vi "CRYPreLoad Project.vi"(4 "Only create refnums (F)":bool) -> ()   [LabVIEW 2013]
uses:
  CRYMainGlobal.vi
  CRYProject Editor Global.vi
  CRYSystem/Program/CRYRef nums global.vi
  CRYSystem/Task Sequence/CRYProject Run Control Global.vi
panel:
  in  "VISA serial ports (empty array)":T1(array[cluster]) {"COM port (1 = COM1, etc.)" min=1 max=99}
  in  "VISA session (for class)":refnum<visa-resource-name>
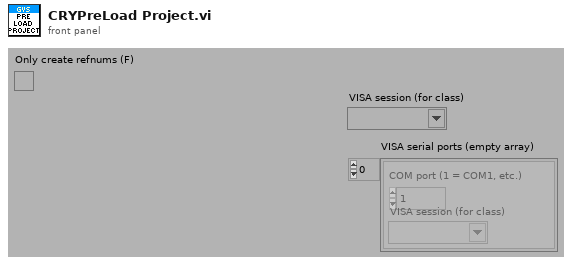
[diagram p1: front panel]
types:
  T1 = cluster{"COM port (1 = COM1, etc.)":i32, "VISA session (for class)":refnum<visa-resource-name>}[]
  T2 = typedef "CRYTS.ctl" = cluster{"No.TS":u16, "TS File Path":path, "TS Name":string, "EditStepName":string, "Steps":T3[], "New State":bool, "Change State":bool, "Flattened CurveLib Data":string, "Document Data":string, "EditStepNo":u16, "Operator Start File":string, "Sequence Type":string, "Sequence Language":string}
  T3 = typedef "CRYStep.ctl" = cluster{"No.VI":i32, "Category":string, "StepName":string, "Seq setup flattened":string, "Comment":string, "Steps config.":bool[], "Jump config":i32[], "Start":dbl, "Increment":dbl, "Name":string, "Unit":string, "Y data":u16, "Y prefix":string, "Y dB ref":dbl, "Y unit":string, "Repeat State Array":cluster{"Start":dbl, "Increment":dbl, "Count":i32, "Num":i32}[]}
  T4 = typedef "CRYHardware.ctl" = cluster{"Name":string, "Analog I/O":u16, "Digital I/O":u16, "Channels":u8, "Dig Dev ID":u8, "N ports":u8, "Interface":u32, "Dig I/O Ports":cluster{"port #":i16, "width":i16, "direction":i32}[], "Interf settings":cluster{"Type":u16, "COM Port":u8, "Baud rate":u32, "Data bits":u32, "Parity":u16, "Stop bits":u16, "Flow control":u16, "Dev ID IEEE":u8}[], "N interfs":i32, "udev SNs":i16[], "udev enable":bool, "Channel Array":T5[], "Cal sequence":string, "SelectedIn":u16, "SelectedOut":u16, "SelectedTab":u16, "State":bool, "Help":string, "Advanced":bool, "In Audio Driver":u16, "Out Audio Driver":u16}
  T5 = typedef "CRYHardware Channel Info.ctl" = cluster{"ID":i32, "Name":string, "Digital":bool, "Input":bool, "Device Name":string, "Hardware Ch ID":u8, "Vmax (V)":dbl, "Latency (samples)":dbl, "Sampling Rate (Hz)":u32, "Bit Depth":u32, "Anti-aliasing Factor (%fs)":sgl, "DAQmx Channel":tag, "term config":i32, "Coupling":i32, "IEPE en":bool, "ASIOChannel Name":string, "Audio Driver":u16, "ASIOChannel Index":u8}
  T6 = cluster{"port #":i16, "width":i16, "direction":i32}[]
  T7 = cluster{"Type":u16, "COM Port":u8, "Baud rate":u32, "Data bits":u32, "Parity":u16, "Stop bits":u16, "Flow control":u16, "Dev ID IEEE":u8}[]
  T8 = typedef "CRYStart Cluster.ctl" = cluster{"SequenceName":string, "Preload Stimulus":bool, "CloseOpenedDisplay":bool, "ClearMeasuredData":bool, "UpdateDisplayDuringRun":bool, "DisplayForConfirmation":bool, "HaltOnFail":bool, "UseSameHardware":bool, "UseSameCalibration":bool}
  T9 = cluster{"DIO Port Config":refnum<vi>, "DIO Port Write":refnum<vi>, "DIO Port Read":refnum<vi>}
  T10 = cluster{"input XON/XOFF":bool, "input HW Handshake":bool, "input alt HW HShk":bool, "output XON/XOFF":bool, "output HW Handshake":bool, "output alt HW HShk":bool, "XOFF byte":u8, "XON byte":u8, "parity error byte":u16}
  T11 = cluster{i32, "VISA session (for class)":refnum<visa-resource-name>}
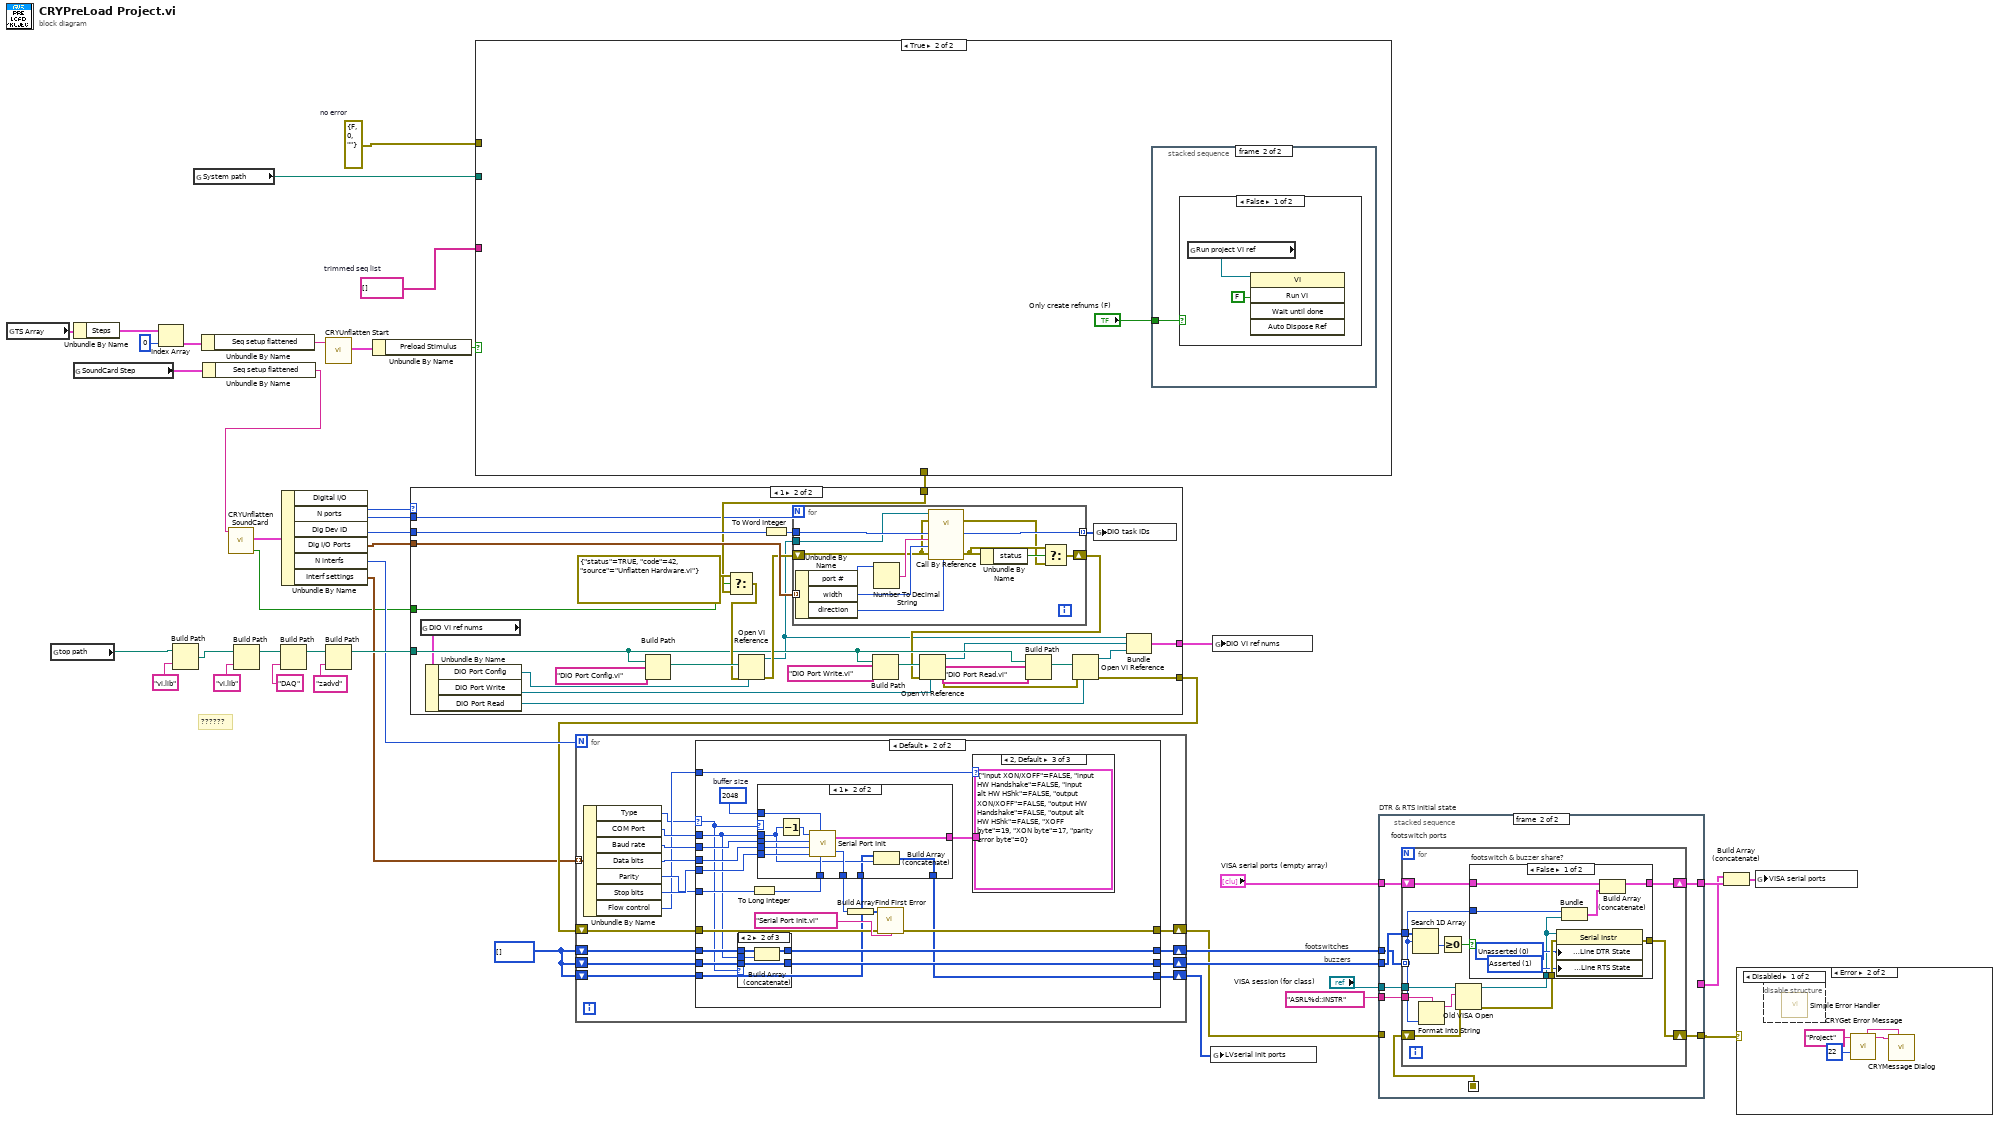
[diagram p0: block diagram]
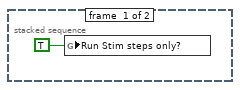
[diagram p5: hidden frame]
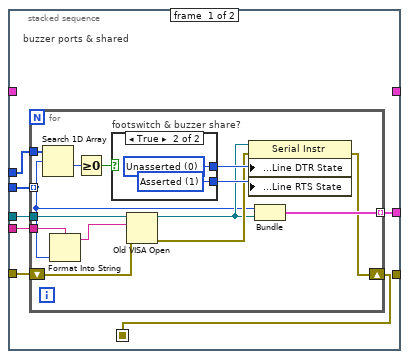
[diagram p7: hidden frame]
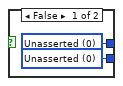
[diagram p8: hidden frame]
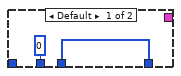
[diagram p11: hidden frame]
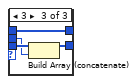
[diagram p13: hidden frame]
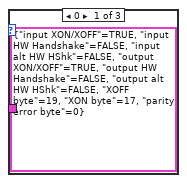
[diagram p14: hidden frame]
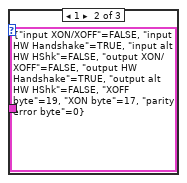
[diagram p15: hidden frame]
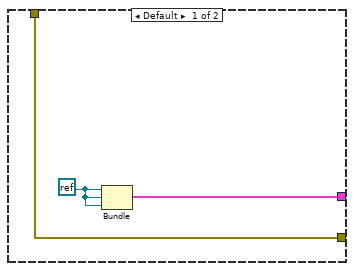
[diagram p16: hidden frame]
diagram:
  w11 = string[] []  # trimmed seq list
  w20 = i32[] []
  w42 = errorcluster {"status"=FALSE, "code"=0, "source"=""}  # no error
  # "??????"
  # "buzzers"
  # "footswitches"
  n1 = global read "CRYProject Editor Global.vi" "TS Array"() -> (w3:T2)
  n2 = global read "CRYMainGlobal.vi" "top path"() -> (w6:path)
  n3 = Unbundle By Name(w3) -> ("Steps"=w2:T3[])
  n4 = global read "CRYProject Editor Global.vi" "SoundCard Step"() -> (w10:T3)
  n5 = Index Array(array=w2, index=0) -> (element=w4:T3)
  n6 = Build Path(base path=w6, name or relative path="vi.lib") -> (appended path=w5:path)
  n7 = global read "CRYMainGlobal.vi" "System path"() -> (w32:path)
  n8 = Unbundle By Name(w4) -> ("Seq setup flattened"=w14:string)
  n9 = Unbundle By Name(w10) -> ("Seq setup flattened"=w9:string)
  n10 = call "CRYUnflatten SoundCard.vi"("Flatten SoundCard"=w9) -> ("Error?"=w17:bool, "SoundCard"=w18:T4)  [unwired: 8 in, 1 out]
  n11 = Build Path(base path=w5, name or relative path="vi.lib") -> (appended path=w34:path)
  n12 = Build Path(base path=w34, name or relative path="DAQ") -> (appended path=w36:path)
  n13 = Unbundle By Name(w18) -> ("Digital I/O"=w39:u16, "N ports"=w40:u8, "Dig Dev ID"=w44:u8, "Dig I/O Ports"=w43:T6, "N interfs"=w31:i32, "Interf settings"=w29:T7)
  n14 = call "CRYUnflatten Start.vi"("Unflatten Sequence"=w14) -> ("Sequence Configure"=w13:T8)  [unwired: 8 in, 2 out]
  n15 = Build Path(base path=w36, name or relative path="zadvd") -> (appended path=w38:path)
  n16 = Unbundle By Name(w13) -> ("Preload Stimulus"=w12:bool)
  n17 = case shown="True" w12 {
    tunnel: [w45 _] -> w41
    tunnel: w42 -> [w45 _]
    tunnel: w32 -> [_ _]
    tunnel: w11 -> [_ _]
    frame False {
    }
    frame True {
      n18 = stacked-sequence {
        tunnel: "Only create refnums (F)" -> [_ w48]
        frame #0 {
          n19 = global write "CRYProject Run Control Global.vi" "Run Stim steps only?"(TRUE ("Run Stim steps only?")) -> ()
        }
        frame #1 {
          n20 = case shown="False" w48 {
            frame False {
              n21 = global read "CRYRef nums global.vi" "Run project VI ref"() -> (w50:refnum<vi>)
              n22 = invoke class="VI" method="Run VI"(reference=w50, "Wait until done"=FALSE ("Wait Until Done")) -> ()  [unwired: 3 in, 5 out]
            }
            frame True {
            }
          }
        }
      }
    }
  }
  n23 = case shown="1" w39 {
    tunnel: w44 -> [_ w81]
    tunnel: w43 -> [_ w78]
    tunnel: w41 -> [w53 w77]
    tunnel: w40 -> [_ w76]
    tunnel: w17 -> [_ w75]
    tunnel: [w53 w60] -> w30
    tunnel: w38 -> [_ w66]
    tunnel: [w51 w56] -> w16
    frame Default {
      w52 = refnum<k0> refnum
      n24 = Bundle(w52, w52, w52) -> (w51:cluster{refnum<k0>, refnum<k0>, refnum<k0>})  [unwired: 1 in]
    }
    frame 1 {
      n25 = global read "CRYRef nums global.vi" "DIO VI ref nums"() -> (w54:T9)
      n26 = Unbundle By Name(w54) -> ("DIO Port Config"=w63:refnum<vi>, "DIO Port Write"=w64:refnum<vi>, "DIO Port Read"=w65:refnum<vi>)
      n27 = Build Path(base path=w66, name or relative path="DIO Port Config.vi") -> (appended path=w73:path)
      n28 = Select(t=errorcluster {"status"=TRUE, "code"=42, "source"="Unflatten Hardware.vi"}, s=w75, f=w77) -> (s? t:f=w72:errorcluster)
      n29 = Open VI Reference(type specifier VI Refnum (for type only)=w63, vi path=w73, error in (no error)=w72) -> (vi reference=w59:refnum<vi>, error out=w71:errorcluster)  [unwired: 3 in]
      n30 = To Word Integer(number=w81) -> (16bit integer=w80:i16)
      n31 = for {
        N: w76 -> [_]
        tunnel: w80 -> [w91]
        shift-right: [w84] -> w62
        shift-left: w71 -> [w86]
        tunnel: w78 -> [w94] mode=indexing
        tunnel: [w92] -> w55 mode=indexing
        tunnel: w59 -> [w87]
        n32 = Unbundle By Name(w94) -> ("port #"=w93:i16, "width"=w89:i16, "direction"=w88:i32)
        n33 = Number To Decimal String(number=w93) -> (decimal integer string=w90:string)  [unwired: 1 in]
        n34 = call-by-ref "?"(reference=w87, error in=w86, "line direction map"=w88, "error in (no error)"=w86, "port width"=w89, "digital channel"=w90, "device"=w91) -> (error out=w82:errorcluster, "error out"=w83:errorcluster, "task ID out"=w92:u32)  [unwired: 5 in, 1 out]
        n35 = Unbundle By Name(w83) -> ("status"=w85:bool)
        n36 = Select(t=w83, s=w85, f=w82) -> (s? t:f=w84:errorcluster)
      }
      n37 = Build Path(base path=w66, name or relative path="DIO Port Write.vi") -> (appended path=w68:path)
      n38 = Open VI Reference(type specifier VI Refnum (for type only)=w64, vi path=w68, error in (no error)=w62) -> (vi reference=w58:refnum<vi>, error out=w61:errorcluster)  [unwired: 3 in]
      n39 = Build Path(base path=w66, name or relative path="DIO Port Read.vi") -> (appended path=w67:path)
      n40 = Open VI Reference(type specifier VI Refnum (for type only)=w65, vi path=w67, error in (no error)=w61) -> (vi reference=w57:refnum<vi>, error out=w60:errorcluster)  [unwired: 3 in]
      n41 = global write "CRYRef nums global.vi" "DIO task IDs"(w55) -> ()
      n42 = Bundle("DIO Port Config"=w59, "DIO Port Write"=w58, "DIO Port Read"=w57) -> (w56:T9)  [unwired: 1 in]
    }
  }
  n43 = for {
    N: w31 -> [_]
    shift-right: [w109] -> w24
    shift-left: w30 -> [w110]
    tunnel: w29 -> [w108] mode=indexing
    shift-right: [w98] -> w27
    shift-left: w20 -> [w101]
    shift-right: [w97] -> w28
    shift-left: w20 -> [w100]
    shift-right: [w95] -> w19
    shift-left: w20 -> [w96]
    n44 = Unbundle By Name(w108) -> ("Type"=w99:u16, "COM Port"=w107:u8, "Baud rate"=w106:u32, "Data bits"=w105:u32, "Parity"=w103:u16, "Stop bits"=w104:u16, "Flow control"=w102:u16)
    n45 = case shown="Default" w99 {
      selector: w99 -> [_ w115]
      tunnel: w110 -> [w114 w131]
      tunnel: [w114 w130] -> w109
      tunnel: w107 -> [_ w118]
      tunnel: w106 -> [_ w129]
      tunnel: w105 -> [_ w128]
      tunnel: w104 -> [_ w127]
      tunnel: w103 -> [_ w126]
      tunnel: w102 -> [_ w125]
      tunnel: w101 -> [w113 w124]
      tunnel: w100 -> [w112 w123]
      tunnel: [w113 w122] -> w98
      tunnel: [w112 w121] -> w97
      tunnel: w96 -> [w111 w117]
      tunnel: [w111 w116] -> w95
      frame 0 {
      }
      frame Default {
        w119 = u16 2048  # buffer size
        n46 = case shown="2" w115 {
          tunnel: [w150 w152 w158] -> w122
          tunnel: w124 -> [w150 w153 w158]
          tunnel: [w149 w154 w155] -> w121
          tunnel: w123 -> [w149 w154 w157]
          tunnel: w118 -> [_ w151 w156]
          frame Default {
          }
          frame 2 {
            n47 = Build Array (concatenate)(w153, w151) -> (w152:i32[])
          }
          frame 3 {
            n48 = Build Array (concatenate)(w157, w156) -> (w155:i32[])
          }
        }
        n49 = To Long Integer(number=w126) -> (32bit integer=w132:i32)
        n50 = case shown="2, Default" w125 {
          tunnel: [T10 {"input XON/XOFF"=TRUE, "input HW Handshake"=FALSE, "input alt HW HShk"=FALSE, "output XON/XOFF"=TRUE, "output HW Handshake"=FALSE, "output alt HW HShk"=FALSE, "XOFF byte"=19, "XON byte"=17, "parity error byte"=0} ("flow control etc.") T10 {"input XON/XOFF"=FALSE, "input HW Handshake"=TRUE, "input alt HW HShk"=FALSE, "output XON/XOFF"=FALSE, "output HW Handshake"=TRUE, "output alt HW HShk"=FALSE, "XOFF byte"=19, "XON byte"=17, "parity error byte"=0} ("flow control etc.") T10 {"input XON/XOFF"=FALSE, "input HW Handshake"=FALSE, "input alt HW HShk"=FALSE, "output XON/XOFF"=FALSE, "output HW Handshake"=FALSE, "output alt HW HShk"=FALSE, "XOFF byte"=19, "XON byte"=17, "parity error byte"=0} ("flow control etc.")] -> w135
          frame 0 {
          }
          frame 1 {
          }
          frame 2, Default {
          }
        }
        n51 = case shown="1" w115 {
          tunnel: w135 -> [_ w148]
          tunnel: w132 -> [_ w147]
          tunnel: w129 -> [_ w146]
          tunnel: w128 -> [_ w145]
          tunnel: w127 -> [_ w144]
          tunnel: [0 ("error code") w143] -> w120
          tunnel: w118 -> [_ w140]
          tunnel: w119 -> [_ w142]
          tunnel: w117 -> [w136 w139]
          tunnel: [w136 w138] -> w116
          frame Default {
          }
          frame 1 {
            n52 = Decrement(x=w140) -> (x-1=w141:u8)
            n53 = call <vilib>:"Serial Port Init.vi"("flow control etc."=w148, "parity"=w147, "buffer size"=w142, "stop bits"=w144, "data bits"=w145, "baud rate"=w146, "port number"=w141) -> ("error code"=w143:i32)
            n54 = Build Array (concatenate)(w139, w140) -> (w138:i32[])
          }
        }
        n55 = Build Array(w120) -> (w134:i32[])
        n56 = call <vilib>:"Find First Error.vi"("error in (no error)"=w131, "source messages"="Serial Port Init.vi", "error codes"=w134) -> ("error out"=w130:errorcluster)  [unwired: 1 in, 1 out]
      }
    }
  }
  n57 = global write "CRYRef nums global.vi" "LVserial init ports"(w19) -> ()
  n58 = global write "CRYRef nums global.vi" "DIO VI ref nums"(w16) -> ()
  n59 = stacked-sequence "DTR & RTS initial state" {
    seq-local: [w163 _] -> [_ w192]
    tunnel: w28 -> [w168 w194]
    tunnel: w27 -> [w167 w193]
    tunnel: "VISA session (for class)" -> [w166 w190]
    tunnel: "ASRL%d::INSTR" -> [w165 w189]
    tunnel: w24 -> [w164 _]
    tunnel: [w162 _] -> w21
    tunnel: [_ w191] -> w8
    tunnel: "VISA serial ports (empty array)" -> [_ w188]
    tunnel: [_ w187] -> w22
    frame #0 {
      # "buzzer ports & shared"
      n60 = for {
        tunnel: w168 -> [w172] mode=indexing
        tunnel: w167 -> [w182]
        tunnel: w166 -> [w178]
        tunnel: w165 -> [w177]
        tunnel: [w171] -> w162 mode=indexing
        shift-right: [w169] -> w163
        shift-left: w164 -> [w170]
        n61 = Search 1D Array(1D array=w182, element=w172) -> (index of element=w181:i32)  [unwired: 1 in]
        n62 = Format Into String(format string=w177, w172) -> (resulting string=w179:string)  [unwired: 2 in, 1 out]
        n63 = Greater Or Equal To 0?(x=w181) -> (x >= 0?=w180:bool)
        n64 = case "footswitch & buzzer share?" shown="True" w180 {
          tunnel: [w184 w186] -> w176
          tunnel: [w183 w185] -> w175
          frame False {
            w184 = i16 0 items=["Unknown"=-1, "Unasserted"=0, "Asserted"=1] ("Modem Line Settings:Line DTR State")
            w183 = i16 0 items=["Unknown"=-1, "Unasserted"=0, "Asserted"=1] ("Modem Line Settings:Line RTS State")
          }
          frame True {
            w186 = i16 0 items=["Unknown"=-1, "Unasserted"=0, "Asserted"=1] ("Modem Line Settings:Line DTR State")
            w185 = i16 1 items=["Unknown"=-1, "Unasserted"=0, "Asserted"=1] ("Modem Line Settings:Line RTS State")
          }
        }
        n65 = Old VISA Open(8:w170, 10:w179, 11:w178) -> (0:w174:errorcluster, 3:w173:refnum<visa-resource-name>)  [unwired: 2 in]
        n66 = property class="Serial Instr"(reference=w173, error in=w174, "Serial Settings:Modem Line Settings:Line DTR State"=w176, "Serial Settings:Modem Line Settings:Line RTS State"=w175) -> (error out=w169:errorcluster)  [unwired: 1 out]
        n67 = Bundle(w172, "VISA session (for class)"=w173) -> (w171:T11)  [unwired: 1 in]
      }
    }
    frame #1 {
      # "footswitch ports"
      n68 = for {
        tunnel: w193 -> [w197] mode=indexing
        tunnel: w194 -> [w207]
        tunnel: w190 -> [w203]
        tunnel: w189 -> [w202]
        shift-right: [w198] -> w191
        shift-left: w192 -> [w201]
        shift-right: [w195] -> w187
        shift-left: w188 -> [w196]
        n69 = Search 1D Array(1D array=w207, element=w197) -> (index of element=w206:i32)  [unwired: 1 in]
        n70 = Format Into String(format string=w202, w197) -> (resulting string=w204:string)  [unwired: 2 in, 1 out]
        n71 = Greater Or Equal To 0?(x=w206) -> (x >= 0?=w205:bool)
        n72 = Old VISA Open(8:w201, 10:w204, 11:w203) -> (0:w199:errorcluster, 3:w200:refnum<visa-resource-name>)  [unwired: 2 in]
        n73 = case "footswitch & buzzer share?" shown="False" w205 {
          tunnel: w200 -> [w211 _]
          tunnel: w199 -> [w216 w218]
          tunnel: [w213 w218] -> w198
          tunnel: w197 -> [w212 _]
          tunnel: w196 -> [w210 w217]
          tunnel: [w209 w217] -> w195
          frame False {
            w215 = i16 0 items=["Unknown"=-1, "Unasserted"=0, "Asserted"=1] ("Modem Line Settings:Line DTR State")
            w214 = i16 1 items=["Unknown"=-1, "Unasserted"=0, "Asserted"=1] ("Modem Line Settings:Line RTS State")
            n74 = property class="Serial Instr"(reference=w211, error in=w216, "Serial Settings:Modem Line Settings:Line DTR State"=w215, "Serial Settings:Modem Line Settings:Line RTS State"=w214) -> (error out=w213:errorcluster)  [unwired: 1 out]
            n75 = Bundle(w212, "VISA session (for class)"=w211) -> (w208:T11)  [unwired: 1 in]
            n76 = Build Array (concatenate)(w210, w208) -> (w209:T1)
          }
          frame True {
          }
        }
      }
    }
  }
  n77 = Build Array (concatenate)(w21, w22) -> (w15:T1)
  n78 = case shown="Error" w8 {
    frame No Error {
    }
    frame Error {
      n79 = disable-structure shown="Disabled" {
        frame Disabled {
          n80 = call <vilib>:"Simple Error Handler.vi"() -> ()  [unwired: 5 in, 5 out]
        }
        frame Enabled {
        }
      }
      n81 = call "CRYGet Error Message.vi"("Error No"=22, "Kind"="Project") -> ("Message"=w219:string, "Window Title"=w220:string)  [unwired: 4 in, 4 out]
      n82 = call "CRYMessage Dialog.vi"("Window Title"=w220, "Message Content"=w219) -> ()  [unwired: 8 in, 2 out]
    }
  }
  n83 = global write "CRYRef nums global.vi" "VISA serial ports"(w15) -> ()
